vi "sub_calculate-covariance.vi"(9 "pw":T1, 10 "px":T1, 11 "x_est":T1) -> (3 "cov":T1)   [LabVIEW 2019]
uses:
  <vilib>/Analysis/Matrix/Datatypes/RealMatrix.ctl
  <vilib>/Analysis/baseanly.llb/Real A x B.vi
  <vilib>/Analysis/Matrix/Numeric/Subtract/Subtract - RM,RM.vi
  <vilib>/Analysis/Matrix/Numeric/Multiply/Multiply - RM,R.vi
  <vilib>/Analysis/Matrix/Numeric/Add/Add - RM,RM.vi
  <vilib>/Analysis/Matrix/Numeric/Subtract/Subtract (Elementwise) - R,RM.vi
  <vilib>/Analysis/Matrix/NI_Matrix.lvlib
  <vilib>/Analysis/NI_AALBase.lvlib
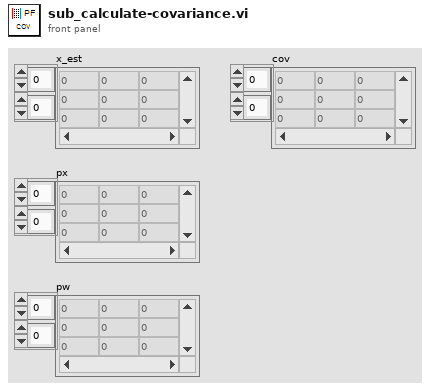
[diagram p1: front panel]
types:
  T1 = typedef "NI_Matrix.lvlib/RealMatrix.ctl" = dbl[][]
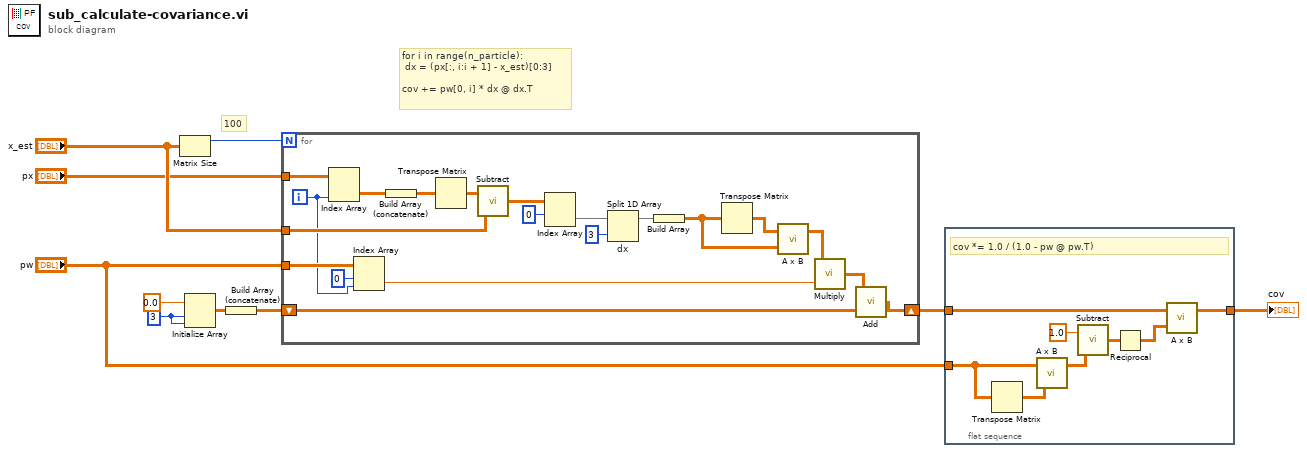
[diagram p0: block diagram]
diagram:
  w2 = 3 ("dimension size")
  # "for i in range(n_particle):\n\tdx = (px[:, i:i + 1] - x_est)[0:3]\n        \ncov += pw[0, i] * dx @ dx.T"
  # "100"
  n1 = Matrix Size(0:"x_est") -> (1:w3:i32)  [unwired: 1 out]
  n2 = Initialize Array(0.0 ("element"), w2, w2) -> (w4:dbl[][])
  n3 = Build Array (concatenate)(w4) -> (w7:T1)
  n4 = for {
    N: w3 -> [_]
    shift-right: [w11] -> w9
    shift-left: w7 -> [w12]
    tunnel: "px" -> [w30]
    tunnel: "x_est" -> [w26]
    tunnel: "pw" -> [w21]
    i -> [w19]
    n5 = Index Array(array=w30, index (col)=w19) -> (element=w29:T1)  [unwired: 1 in]
    n6 = Index Array(array=w21, index (row)=0, index (col)=w19) -> (element=w15:dbl)
    n7 = Build Array (concatenate)(w29) -> (w28:T1)
    n8 = Transpose Matrix(1:w28) -> (0:w27:T1)
    n9 = call-poly <vilib>:"Subtract.vi"("Real Matrix B"=w26, "Real Matrix A"=w27) -> ("A - B"=w25:T1)
    n10 = Index Array(array=w25, index (row)=0) -> (element=w23:dbl[])  [unwired: 1 in]
    n11 = Split 1D Array "dx"(array=w23, index=3) -> (first subarray=w18:dbl[])  [unwired: 1 out]
    n12 = Build Array(w18) -> (w16:T1)
    n13 = Transpose Matrix(1:w16) -> (0:w17:T1)
    n14 = call-poly <vilib>:"A x B.vi"("B"=w16, "A"=w17) -> ("A x B"=w14:T1)  [unwired: 1 out]
    n15 = call-poly <vilib>:"Multiply.vi"("Real Scalar c"=w15, "Real Matrix A"=w14) -> ("A * c"=w13:T1)
    n16 = call-poly <vilib>:"Add.vi"("Real Matrix B"=w12, "Real Matrix A"=w13) -> ("A + B"=w11:T1)
  }
  n17 = flat-sequence {
    tunnel: "pw" -> [w37]
    tunnel: w9 -> [w32]
    tunnel: [w31] -> w10
    frame #0 {
      # "cov *= 1.0 / (1.0 - pw @ pw.T)"
      n18 = Transpose Matrix(1:w37) -> (0:w38:T1)
      n19 = call-poly <vilib>:"A x B.vi"("B"=w38, "A"=w37) -> ("A x B"=w36:T1)  [unwired: 1 out]
      n20 = call-poly <vilib>:"Subtract.vi"("Real Matrix A"=w36, "Real Scalar c"=1.0) -> ("c - A"=w34:T1)
      n21 = Reciprocal(x=w34) -> (1/x=w33:T1)
      n22 = call-poly <vilib>:"A x B.vi"("B"=w33, "A"=w32) -> ("A x B"=w31:T1)  [unwired: 1 out]
    }
  }
  "cov" <- w10
